vi "Clear.vi"(8 "error in (no error)":errorcluster, 11 "Mock Worker In":refnum<class "Mock Worker.lvclass">) -> (0 "error out":errorcluster)   [LabVIEW 2020, in "Mock Worker.lvclass"]
doc: "Clears any resorces allocated during initialization."
uses:
  Mock Worker.lvclass
  <vilib>/Asteme/Triarc Framework/Base/Base.lvclass
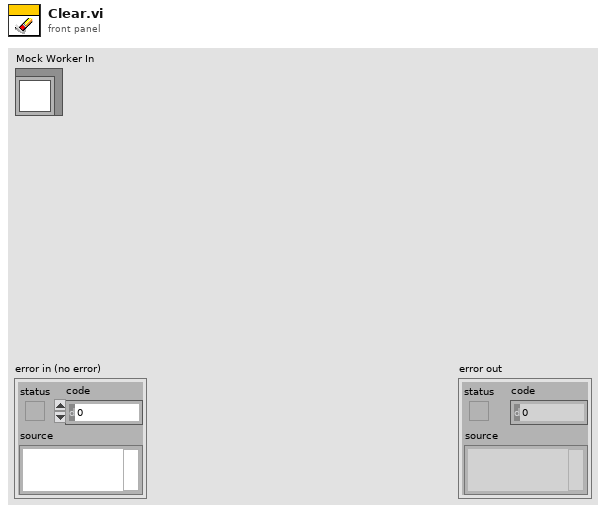
[diagram p1: front panel]
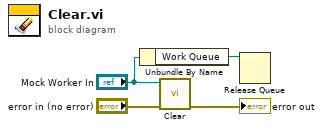
[diagram p0: block diagram]
diagram:
  n1 = Unbundle By Name("Mock Worker In") -> ("Work Queue"=w1:refnum<queue>)
  n2 = call-parent "Clear.vi"("error in (no error)"="error in (no error)", "Base In"="Mock Worker In") -> ("error out"=→"error out":errorcluster)  [unwired: 9 in]
  n3 = Release Queue(queue=w1) -> ()  [unwired: 2 in, 3 out]
